vi "Signal Generator.vi"(0 "Clock in":refnum<k21>, 1 "WG Number":i16, 3 "Enabled":bool) -> ()   [LabVIEW 2013, in "IRIO.lvlib"]
uses:
  IRIO.lvlib
  common/GlobalReg.vi
  <vilib>/Platform/TimedLoop/XDataNode/wakeup.ctl
  <vilib>/Platform/TimedLoop/XDataNode/XDNodeRunTimeDep.lvlib
  <vilib>/Platform/TimedLoop/XDataNode/nitl_modes.ctl
  <vilib>/Platform/TimedLoop/XDataNode/timing_clust.ctl
  <vilib>/Platform/TimedLoop/XDataNode/XDataNode.xnode
  <vilib>/eio/EIONode/EIONode.xnode
  <vilib>/rvi/eio/common/nirviEmuTemplateMethod_errors.vi
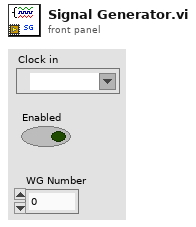
[diagram p1: front panel]
types:
  T1 = typedef "XDNodeRunTimeDep.lvlib/timing_clust.ctl" = cluster{"Expected End [f-1]":u64, "Actual End [f-1]":u64, "Finished Late? [f-1]":bool, "Expected End [i-1]":u64, "Actual End [i-1]":u64, "Finished Late? [i-1]":bool, "Expected Start [i]":u64, "Actual Start [i]":u64, "Expected Start [f]":u64, "Actual Start [f]":u64, "Source Name":string, "Structure Name":string, "Period":i64, "Deadline":i64, "Offset":i64, "Start":i64, "Priority":i32, "Timeout":i32, "Mode":T2, "Wakeup Reason":T3, "Error":errorcluster, "Source Type":string, "Secondary Source Type":string, "Global End Time":u64, "Global Start Time":u64, "Frame Duration":u64, "Iteration Duration":u64, "Assigned CPU":i32, "I/O Scan Engine Mode":u32}
  T2 = typedef "XDNodeRunTimeDep.lvlib/nitl_modes.ctl" = enum32{"No Change", "Process missed periods, maintain original phase", "Discard missed periods, maintain original phase", "Process missed periods, ignore original phase", "Discard missed periods, ignore original phase"}
  T3 = typedef "XDNodeRunTimeDep.lvlib/wakeup.ctl" = enum32{"Normal", "Aborted", "Asynchronous wakeup", "Timing source error", "Timed loop error", "Timeout"}
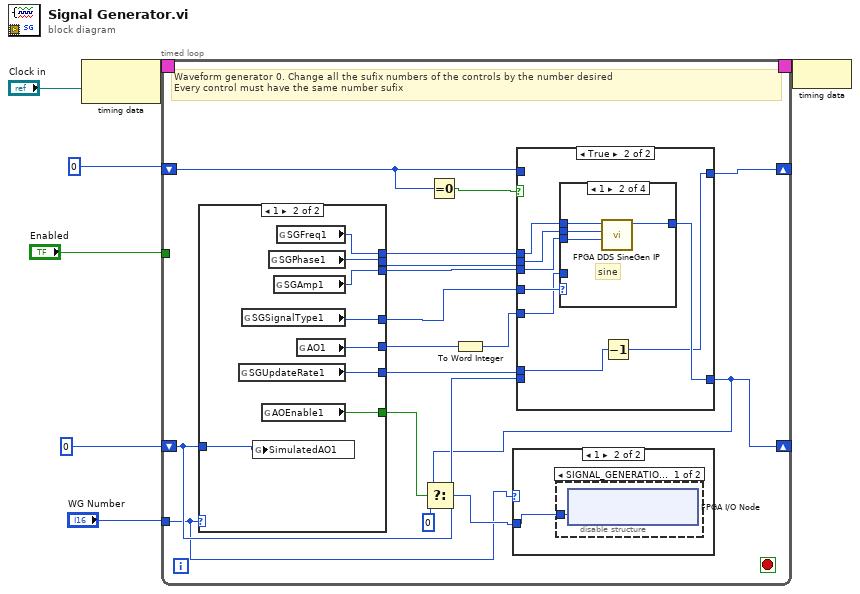
[diagram p0: block diagram]
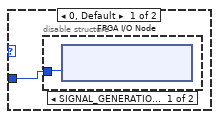
[diagram p2: hidden frame]
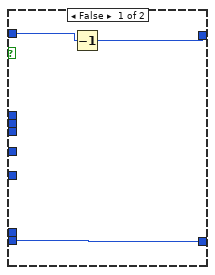
[diagram p5: hidden frame]
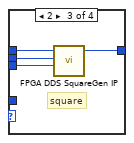
[diagram p7: hidden frame]
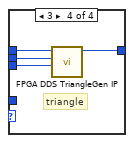
[diagram p8: hidden frame]
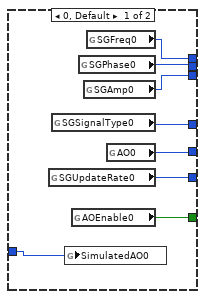
[diagram p9: hidden frame]
diagram:
  n1 = node-c288("Clock in") -> (w7:T1)
  n2 = timed-loop {
    shift-right: [w11] -> _
    shift-left: i16 0 ("Signal Value") -> [w18]
    timing: w7 -> [_]
    timing-out: [_] -> w6
    shift-right: [w14] -> _
    shift-left: u32 0 -> [w13]
    tunnel: "Enabled" -> [_]
    tunnel: "WG Number" -> [w8]
    stop <- _ stop-if-true
    # "Waveform generator 0. Change all the sufix numbers of the controls by the number desired\nEvery control must have the same number sufix"
    n3 = case shown="1" w8 {
      tunnel: [w59 w67] -> w23
      tunnel: [w58 w66] -> w22
      tunnel: [w57 w65] -> w21
      tunnel: [w56 w64] -> w12
      tunnel: [w55 w63] -> w20
      tunnel: [w54 w62] -> w15
      tunnel: [w53 w61] -> w19
      tunnel: w18 -> [w52 w60]
      frame 0, Default {
        n4 = global read "GlobalReg.vi" "SGUpdateRate0"() -> (w54:u32)
        n5 = global read "GlobalReg.vi" "SGSignalType0"() -> (w55:u8)
        n6 = global write "GlobalReg.vi" "SimulatedAO0"(w52) -> ()
        n7 = global read "GlobalReg.vi" "AOEnable0"() -> (w56:bool)
        n8 = global read "GlobalReg.vi" "SGPhase0"() -> (w58:u32)
        n9 = global read "GlobalReg.vi" "SGAmp0"() -> (w57:u16)
        n10 = global read "GlobalReg.vi" "SGFreq0"() -> (w59:u32)
        n11 = global read "GlobalReg.vi" "AO0"() -> (w53:i32)
      }
      frame 1 {
        n12 = global read "GlobalReg.vi" "SGUpdateRate1"() -> (w62:u32)
        n13 = global read "GlobalReg.vi" "SGSignalType1"() -> (w63:u8)
        n14 = global write "GlobalReg.vi" "SimulatedAO1"(w60) -> ()
        n15 = global read "GlobalReg.vi" "AOEnable1"() -> (w64:bool)
        n16 = global read "GlobalReg.vi" "SGPhase1"() -> (w66:u32)
        n17 = global read "GlobalReg.vi" "SGAmp1"() -> (w65:u16)
        n18 = global read "GlobalReg.vi" "SGFreq1"() -> (w67:u32)
        n19 = global read "GlobalReg.vi" "AO1"() -> (w61:i32)
      }
    }
    n20 = Equal To 0?(x=w13) -> (x = 0?=w16:bool)
    n21 = To Word Integer(number=w19) -> (16bit integer=w17:i16)
    n22 = case shown="True" w16 {
      tunnel: w23 -> [_ w38]
      tunnel: w22 -> [_ w37]
      tunnel: w21 -> [_ w36]
      tunnel: [w30 w35] -> w11
      tunnel: w20 -> [_ w34]
      tunnel: w17 -> [_ w33]
      tunnel: w18 -> [w30 _]
      tunnel: w15 -> [_ w32]
      tunnel: [w28 w31] -> w14
      tunnel: w13 -> [w29 _]
      frame False {
        n23 = Decrement(x=w29) -> (x-1=w28:u32)
      }
      frame True {
        n24 = case shown="1" w34 {
          tunnel: w38 -> [_ w43 w47 w51]
          tunnel: w37 -> [_ w42 w46 w50]
          tunnel: w36 -> [_ w41 w45 w49]
          tunnel: [w39 w40 w44 w48] -> w35
          tunnel: w33 -> [w39 _ _ _]
          frame 0, Default {
          }
          frame 1 {
            # "sine"
            n25 = call "FPGA DDS SineGen IP.vi"("Signal Amplitude (x 2^15)"=w41, "Phase Shift"=w42, "Accumulator Increment"=w43) -> ("Signal Value"=w40:i16)  [unwired: 7 in, 1 out]
          }
          frame 2 {
            # "square"
            n26 = call "FPGA DDS SquareGen IP.vi"("Signal Amplitude (x 2^15)"=w45, "Phase Shift"=w46, "Accumulator Increment"=w47) -> ("Signal Value"=w44:i16)  [unwired: 7 in, 1 out]
          }
          frame 3 {
            # "triangle"
            n27 = call "FPGA DDS TriangleGen IP.vi"("Signal Amplitude (x 2^15)"=w49, "Phase Shift"=w50, "Accumulator Increment"=w51) -> ("Signal Value"=w48:i16)  [unwired: 7 in, 1 out]
          }
        }
        n28 = Decrement(x=w32) -> (x-1=w31:u32)
      }
    }
    n29 = Select(t=w11, s=w12, f=i16 0) -> (s? t:f=w9:i16)
    n30 = case shown="1" w8 {
      tunnel: w9 -> [w24 w26]
      frame 0, Default {
        n31 = disable-structure shown="SIGNAL_GENERATION_SIMULATED==NO, Default" {
          disable-tunnel: w24 -> [w25 _]
          frame condition #0 (active) {
            n32 = xnode "FPGA I/O Node"("IO Module\\AO 0"=w25) -> ()  [unwired: 1 in, 1 out]
          }
          frame condition #1 {
          }
        }
      }
      frame 1 {
        n33 = disable-structure shown="SIGNAL_GENERATION_SIMULATED==NO, Default" {
          disable-tunnel: w26 -> [w27 _]
          frame condition #0 (active) {
            n34 = xnode "FPGA I/O Node"("IO Module\\AO 1"=w27) -> ()  [unwired: 1 in, 1 out]
          }
          frame condition #1 {
          }
        }
      }
    }
  }
  n35 = node-c288(w6) -> ()
